vi "generate UI user event.vi"(11 "Template in":refnum<class "Template.lvclass">) -> (3 "Template out":refnum<class "Template.lvclass">)   [LabVIEW 2020, in "Template.lvlib" / "Template.lvclass"]
uses:
  Template.lvclass
  Template.lvclass/Template.ctl
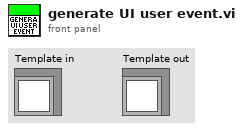
[diagram p1: front panel]
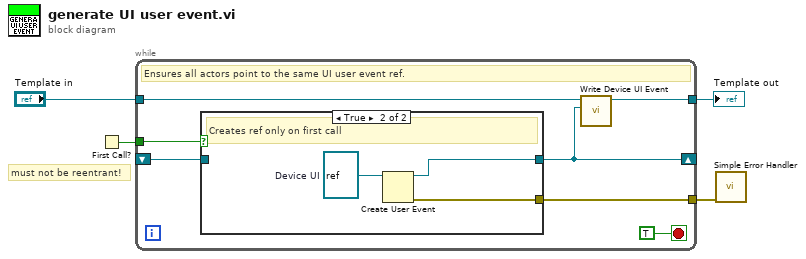
[diagram p0: block diagram]
diagram:
  # "must not be reentrant!"
  n1 = First Call?() -> (First Call?: T/F=w2:bool)
  n2 = while {
    tunnel: [w11] -> w1
    tunnel: w2 -> [w7]
    tunnel: "Template in" -> [w6]
    tunnel: [w9] -> w3
    shift-right: [w5] -> _
    shift-left: _ -> [w8]
    stop <- TRUE stop-if-true
    # "Ensures all actors point to the same UI user event ref."
    n3 = case shown="True" w7 {
      tunnel: [_ w15] -> w11
      tunnel: [w12 w14] -> w5
      tunnel: w8 -> [w12 _]
      frame False {
        # "Not first call. Use created ref."
      }
      frame True {
        w13 = refnum<vi> refnum  # Device UI
        # "Creates ref only on first call"
        n4 = Create User Event(user event datatype=w13) -> (user event=w14:refnum<user-event>, error out=w15:errorcluster)  [unwired: 1 in]
      }
    }
    n5 = call "Write Device UI Event.vi"("Device UI Event"=w5, "Template in"=w6) -> ("Template out"=w9:refnum<class "Template.lvclass">)  [unwired: 9 in]
  }
  "Template out" <- w3
  n6 = call <vilib>:"Simple Error Handler.vi"("error in (no error)"=w1) -> ()  [unwired: 4 in, 5 out]
